vi "Run Bfr Rx - Handle Offset.vi"(7 "Offset in":u64, 8 "error in (no error)":errorcluster, 9 "Buffer Size":i32, 10 "Data":u8[](array[numeric])) -> (0 "error out":errorcluster, 2 "Data Size":i32, 5 "Offset out":u64)   [LabVIEW 2016, in "UDP-Custom-Device Engine.lvlib"]
uses:
  UDP-Custom-Device Engine.lvlib
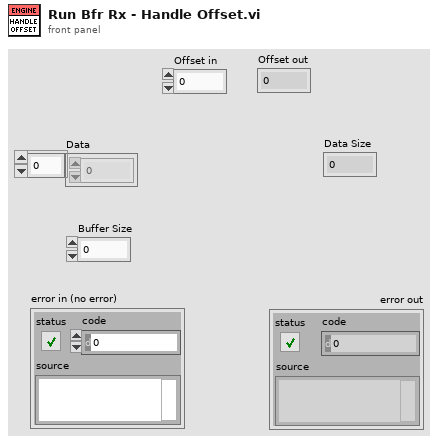
[diagram p1: front panel]
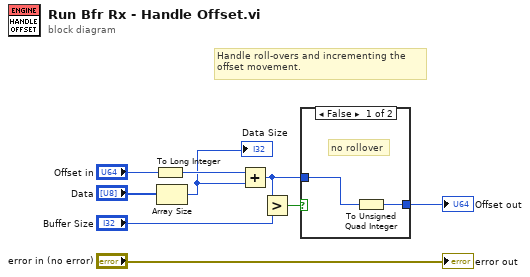
[diagram p0: block diagram]
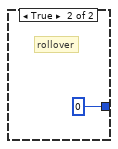
[diagram p2: hidden frame]
diagram:
  # "Handle roll-overs and incrementing the\noffset movement."
  n1 = To Long Integer(number="Offset in") -> (32bit integer=w4:i32)
  n2 = Array Size(array="Data") -> (size(s)=w3:i32)
  "Data Size" <- w3
  n3 = Add(x=w4, y=w3) -> (x+y=w2:i32)
  n4 = Greater?(x=w2, y="Buffer Size") -> (0:w6:bool)
  n5 = case shown="False" w6 {
    tunnel: [w11 u64 0 ("Offset out")] -> w5
    tunnel: w2 -> [w10 _]
    frame False {
      # "no rollover"
      n6 = To Unsigned Quad Integer(1:w10) -> (0:w11:u64)
    }
    frame True {
      # "rollover"
    }
  }
  "Offset out" <- w5
  "error out" <- "error in (no error)"
